vi "MFCevaluation.vi"(5 "MFCcapabilities":T2[](array[typedef]), 8 "MdotRequest":dbl) -> (1 "EvaluatedMFCs":T1[](array[typedef]) {"OffsetFromCentre" format="%#.2f"; "RangeFraction" format="%#_3f"})   [LabVIEW 2016]
uses:
  MFCcapability.ctl
  MFCevaluation.ctl
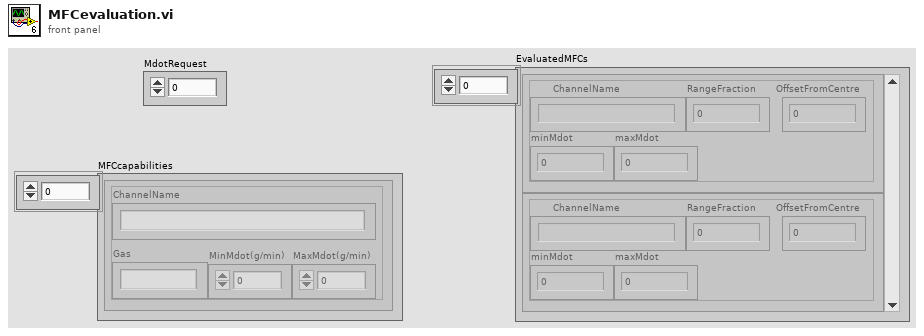
[diagram p1: front panel]
types:
  T1 = typedef "MFCevaluation.ctl" = cluster{"OffsetFromCentre":dbl, "ChannelName":string, "RangeFraction":dbl, "minMdot":dbl, "maxMdot":dbl}
  T2 = typedef "MFCcapability.ctl" = cluster{"ChannelName":string, "MinMdot(g/min)":dbl, "MaxMdot(g/min)":dbl, "Gas":string}
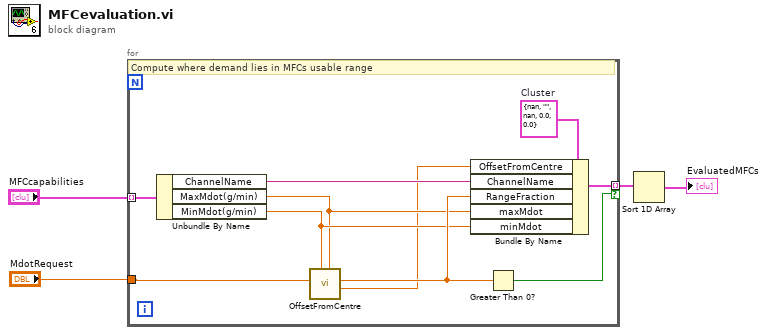
[diagram p0: block diagram]
diagram:
  n1 = for {
    tunnel: "MdotRequest" -> [w5]
    tunnel: "MFCcapabilities" -> [w14] mode=indexing
    tunnel: [w12] -> w2 mode=indexing if=w11
    w9 = T1 {"OffsetFromCentre"=nan, "ChannelName"="", "RangeFraction"=nan, "minMdot"=0.0, "maxMdot"=0.0}  # Cluster
    # "Compute where demand lies in MFCs usable range"
    n2 = Unbundle By Name(w14) -> ("ChannelName"=w13:string, "MaxMdot(g/min)"=w7:dbl, "MinMdot(g/min)"=w8:dbl)
    n3 = call "OffsetFromCentre.vi"("RangeMax"=w7, "RangeMin"=w8, "Value"=w5) -> ("OffsetFromCentre"=w6:dbl, "LocationInRange"=w10:dbl)  [unwired: 6 in, 1 out]
    n4 = Bundle By Name(cluster=w9, "OffsetFromCentre"=w6, "ChannelName"=w13, "RangeFraction"=w10, "maxMdot"=w7, "minMdot"=w8) -> (w12:T1)
    n5 = Greater Than 0?(x=w10) -> (x > 0?=w11:bool)
  }
  n6 = Sort 1D Array(array=w2) -> (sorted array=→"EvaluatedMFCs":T1[])
